vi "LoadMainPanel.vi"(8 "error in (no error)":errorcluster, 11 "MPC_VirbVision in":refnum<class "MPC_VirbVision.lvclass">) -> (0 "error out":errorcluster, 2 "This VI":refnum<vi>, 3 "MPC_VirbVision out":refnum<class "MPC_VirbVision.lvclass">)   [LabVIEW 2019, in "MPC_VirbVision.lvclass"]
uses:
  MPC_VirbVision.lvclass
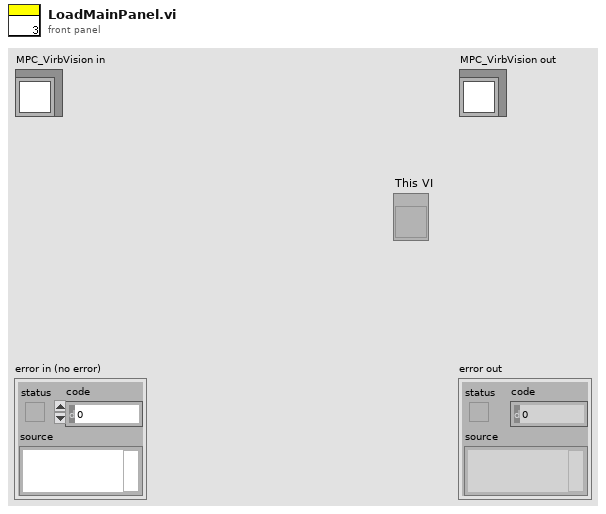
[diagram p1: front panel]
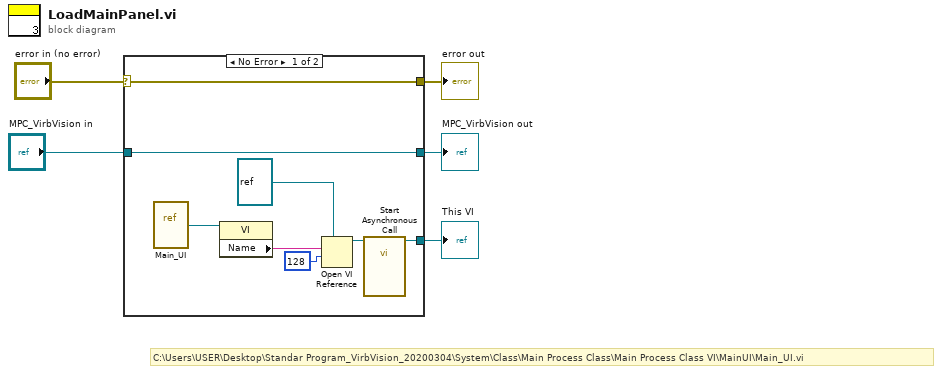
[diagram p0: block diagram]
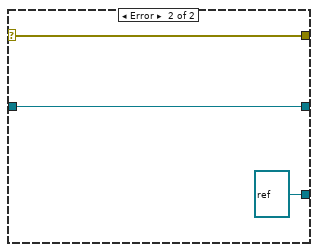
[diagram p2: hidden frame]
diagram:
  # "C:\\Users\\USER\\Desktop\\Standar Program_VirbVision_20200304\\System\\Class\\Main Process Class\\Main Process Class VI\\MainUI\\Main_UI.vi"
  n1 = case shown="No Error" "error in (no error)" {
    selector: "error in (no error)" -> [w8 w14]
    tunnel: "MPC_VirbVision in" -> [w6 w16]
    tunnel: [w6 w16] -> w3
    tunnel: [w9 refnum<vi> refnum ("type specifier VI Refnum (for type only)")] -> w2
    tunnel: [w8 w14] -> w1
    frame No Error {
      n2 = vi-ref "Main_UI.vi"() -> (w7:refnum<vi>)
      n3 = property class="VI"(reference=w7) -> ("Name"=w10:string)  [unwired: 1 in, 2 out]
      n4 = Open VI Reference(type specifier VI Refnum (for type only)=refnum<vi> refnum, vi path=w10, options=128) -> (vi reference=w13:refnum<vi>)  [unwired: 3 in, 1 out]
      n5 = call-by-ref "Start Asynchronous Call"(reference=w13) -> (reference out=w9:refnum<vi>)  [unwired: 12 in, 2 out]
    }
    frame Error {
    }
  }
  "error out" <- w1
  "MPC_VirbVision out" <- w3
  "This VI" <- w2
